vi "getPictureStreamAndInfos.vi"(8 "error in (no error)":errorcluster, 11 "Picture Path":path) -> (0 "error out":errorcluster, 1 "File Name":string, 2 "PictureType":T1 items=["BMP"=11, "DIB"=7, "EMF"=2, "EPS"=10, "GIF"=8, "JPEG"=5, "PICT"=4, "PNG"=6, "TIFF"=9, "WMF"=3, "WPG"=12], 3 "FileStream out":refnum<k24>, 4 "Picture Size":cluster{"width":i32, "height":i32})   [LabVIEW 2017, in "LabVIEW NPOI.lvlib" / "xwpfWriter.lvclass"]
uses:
  xwpfWriter.lvclass
  Picture Type.ctl
  <vilib>/picture/picture.llb/imagedata.ctl
  Support/File Stream/File Stream.lvlib
  LabVIEW NPOI.lvlib
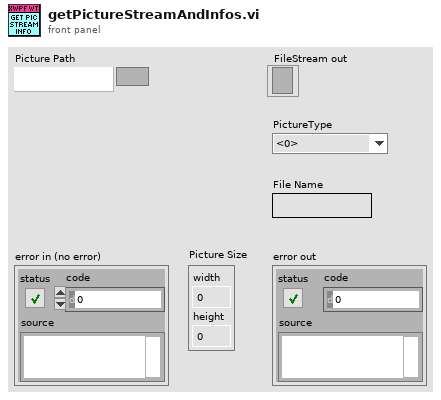
[diagram p1: front panel]
types:
  T1 = typedef "LabVIEW NPOI.lvlib/Picture Type.ctl" = i32
  T2 = typedef "imagedata.ctl" = cluster{"image type":i32, "image depth":i32, "image":u8[], "mask":u8[], "colors":u32[], "Rectangle":cluster{"left":i16, "top":i16, "right":i16, "bottom":i16}}
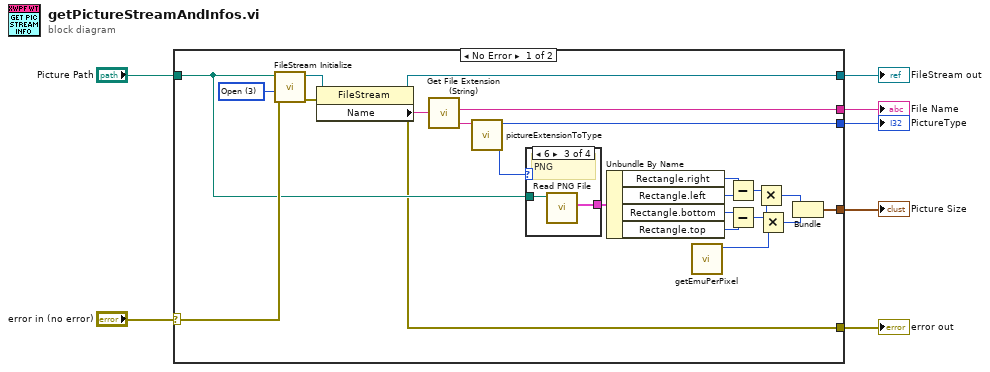
[diagram p0: block diagram]
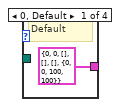
[diagram p2: hidden frame]
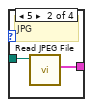
[diagram p3: hidden frame]
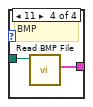
[diagram p4: hidden frame]
diagram:
  n1 = case shown="No Error" "error in (no error)" {
    selector: "error in (no error)" -> [w29 w37]
    tunnel: [w28 _] -> w6
    tunnel: [w27 _] -> w5
    tunnel: "Picture Path" -> [w18 _]
    tunnel: [w17 w37] -> w3
    tunnel: [w14 _] -> w2
    tunnel: [w8 _] -> w1
    frame No Error {
      w13 = 3 items=["CreateNew"=1, "Create"=2, "Open"=3, "OpenOrCreate"=4, "Truncate"=5, "Append"=6] ("mode")
      n2 = call "FileStream Initialize.vi"("error in (no error)"=w29, "mode"=w13, "path"=w18) -> ("error out"=w11:errorcluster, "new reference"=w12:refnum<k24>)  [unwired: 7 in]
      n3 = property class="FileStream"(reference=w12, error in=w11) -> (reference out=w27:refnum<k24>, error out=w17:errorcluster, "Name"=w15:string)
      n4 = call "Get File Extension (String).vi"("File Path"=w15) -> ("File Name"=w14:string, "File Extension"=w16:string)  [unwired: 9 in]
      n5 = call "pictureExtensionToType.vi"("Picture File Extension"=w16) -> ("PictureType"=w28:T1)  [unwired: 10 in]
      n6 = case shown="6" w28 {
        tunnel: w18 -> [_ w32 w34 w36]
        tunnel: [T2 {"image type"=0, "image depth"=0, "image"=[], "mask"=[], "colors"=[], "Rectangle"={"left"=0, "top"=0, "right"=100, "bottom"=100}} ("image data") w31 w33 w35] -> w19
        frame 0, Default {
          # "Default"
        }
        frame 5 {
          # "JPG"
          n7 = call <vilib>:"Read JPEG File.vi"("path to JPEG file"=w32) -> ("image data"=w31:T2)  [unwired: 8 in, 2 out]
        }
        frame 6 {
          # "PNG"
          n8 = call <vilib>:"Read PNG File.vi"("path to PNG file"=w34) -> ("image data"=w33:T2)  [unwired: 8 in, 2 out]
        }
        frame 11 {
          # "BMP"
          n9 = call <vilib>:"Read BMP File.vi"("path to BMP file"=w36) -> ("image data"=w35:T2)  [unwired: 8 in, 2 out]
        }
      }
      n10 = Unbundle By Name(w19) -> ("Rectangle.right"=w21:i16, "Rectangle.left"=w20:i16, "Rectangle.bottom"=w22:i16, "Rectangle.top"=w23:i16)
      n11 = call "getEmuPerPixel.vi"() -> ("EMU_PER_PIXEL"=w26:i32)  [unwired: 10 in, 1 out]
      n12 = Subtract(x=w21, y=w20) -> (x-y=w24:i16)
      n13 = Subtract(x=w22, y=w23) -> (x-y=w25:i16)
      n14 = Multiply(x=w24, y=w26) -> (x*y=w10:i32)
      n15 = Multiply(x=w25, y=w26) -> (x*y=w9:i32)
      n16 = Bundle(w10, w9) -> (w8:cluster{i32, i32})  [unwired: 1 in]
    }
    frame Error {
    }
  }
  "PictureType" <- w6
  "FileStream out" <- w5
  "error out" <- w3
  "File Name" <- w2
  "Picture Size" <- w1
